vi "Finalización_BIn.vi"(0 "Refnum in":refnum<k21>, 5 "error in (no error)":errorcluster) -> (19 "error out":errorcluster)   [LabVIEW 2013]
uses:
  <vilib>/DAQmx/write.llb/DAQmx Write (Digital U32 1Chan 1Samp).vi
  <vilib>/DAQmx/miscellaneous.llb/DAQmx Fill In Error Info.vi
panel:
  out "number":u32
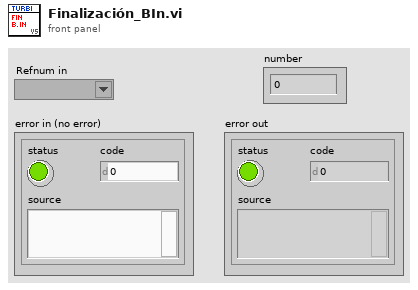
[diagram p1: front panel]
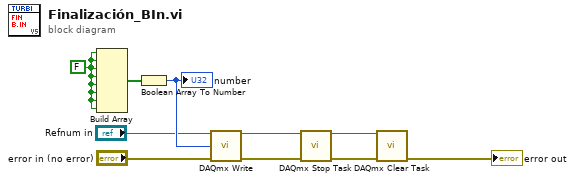
[diagram p0: block diagram]
diagram:
  w8 = FALSE
  n1 = Build Array(w8, w8, w8, w8, w8, w8, w8, w8) -> (w9:bool[])
  n2 = Boolean Array To Number(Boolean array=w9) -> (number=w10:u32)
  "number" <- w10
  n3 = call-poly <vilib>:"DAQmx Write.vi"("task/channels in"="Refnum in", "data"=w10, "error in"="error in (no error)") -> ("task out"=w4:refnum<k21>, "error out"=w5:errorcluster)  [unwired: 10 in, 1 out]
  n4 = call <vilib>:"DAQmx Stop Task.vi"("task/channels in"=w4, "error in"=w5) -> ("task out"=w2:refnum<k21>, "error out"=w3:errorcluster)  [unwired: 12 in]
  n5 = call <vilib>:"DAQmx Clear Task.vi"("task in"=w2, "error in"=w3) -> ("error out"=→"error out":errorcluster)  [unwired: 13 in]
